vi "02 Blinking LEDs.vi"() -> ()   [LabVIEW 2019]
panel:
  in  "milliseconds to wait":u32=500
  out "LEDs":bool[](array[boolean])
  # "Hit Cmd E to see the diagram (code)"
  # "Can you:\n1. change the speed of the moving light?  Make it faster or slower?\n2. make it go to 16 different slots?\n3. make it go to 32 slots?\n4. make the LEDs red rather than green?\n5. the LED movement cycles forever through the array\n6. change the code so that once the LED is turned on it stays on\n7. have two LED strings, one that keeps old ones on and the other that does not?"
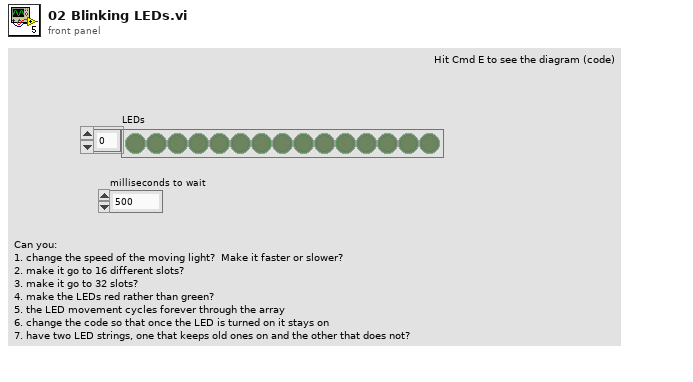
[diagram p1: front panel]
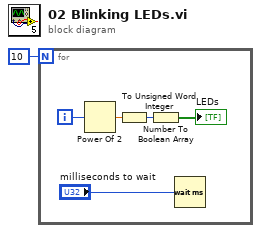
[diagram p0: block diagram]
diagram:
  n1 = for {
    N: 10 -> [_]
    i -> [w6]
    n2 = Power Of 2(x=w6) -> (2^x=w5:dbl)
    n3 = To Unsigned Word Integer(number=w5) -> (unsigned 16bit integer=w2:u16)
    n4 = Number To Boolean Array(number=w2) -> (Boolean array=→"LEDs":bool[])
    n5 = Wait (ms)(milliseconds to wait="milliseconds to wait") -> ()  [unwired: 1 out]
  }
